vi "To Catalogue Cluster.vi"(8 "error in":errorcluster, 10 "Raw Catalogue":string="DEV:DB3.L1:LVL:DEV:MB1.T1:TEMP:DEV:DB7.G1:AUX:DEV:MB0.H1:HTR\n") -> (0 "error out":errorcluster, 1 "Devices":string[](array[string]), 2 "Catalouge":T1)   [LabVIEW 2015, in "Mercury iXX.lvlib"]
uses:
  Mercury iXX.lvlib
  Public/Libraries/System/Controls/Catalogue.ctl
  <vilib>/regexp/Match Regular Expression.xnode
  Public/Libraries/System.lvlib
panel:
  # "Mainboard"
  # "Daughter Boards"
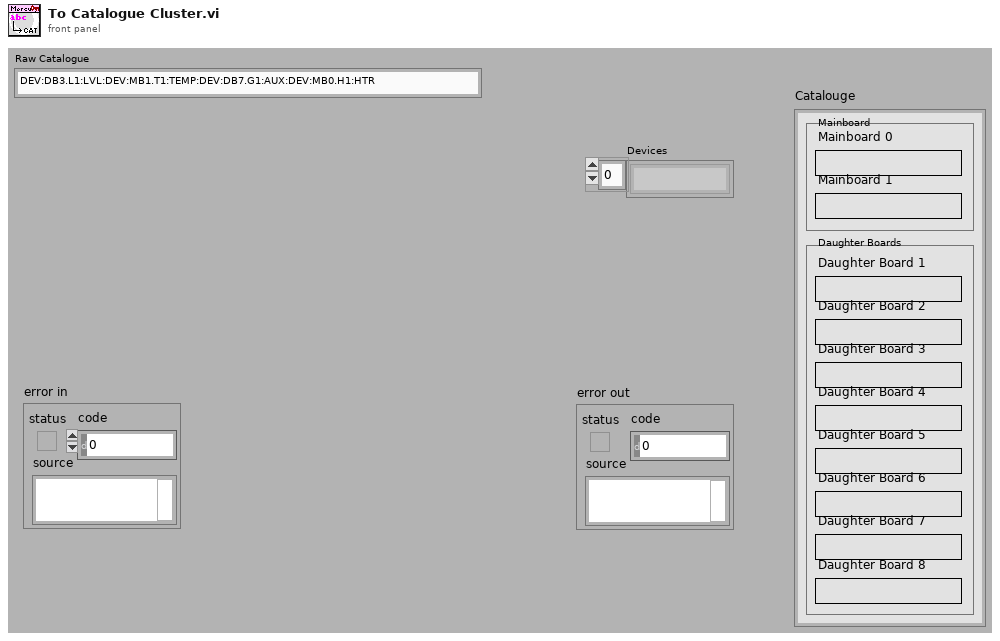
[diagram p1: front panel]
types:
  T1 = typedef "Mercury iXX.lvlib/System.lvlib/Catalogue.ctl" = cluster{"Mainboard 0":string, "Mainboard 1":string, "Daughter Board 1":string, "Daughter Board 2":string, "Daughter Board 3":string, "Daughter Board 4":string, "Daughter Board 5":string, "Daughter Board 6":string, "Daughter Board 7":string, "Daughter Board 8":string}
  T2 = cluster{"[0]":string, "[1]":string, "[2]":string, "[3]":string, "[4]":string, "[5]":string, "[6]":string, "[7]":string, "[8]":string, "[9]":string}
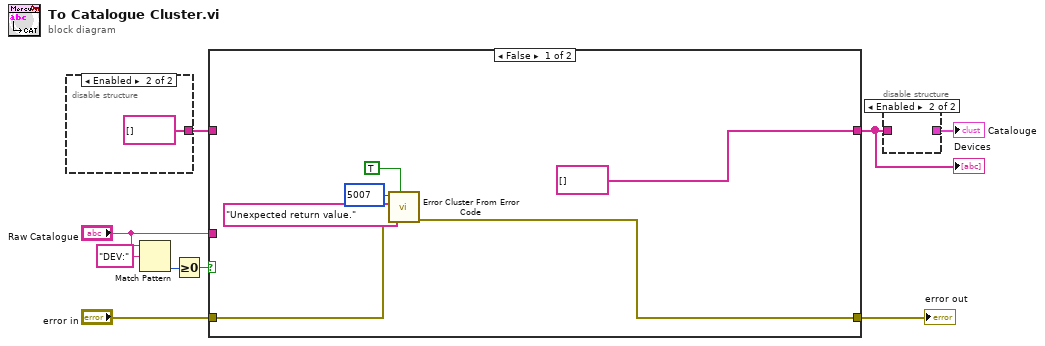
[diagram p0: block diagram]
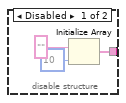
[diagram p2: hidden frame]
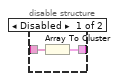
[diagram p3: hidden frame]
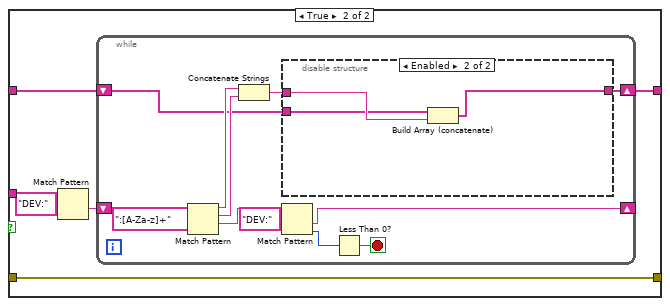
[diagram p4: hidden frame]
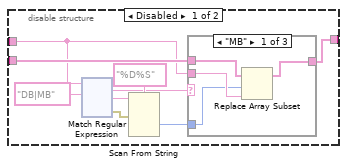
[diagram p5: hidden frame]
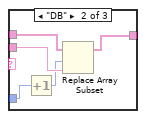
[diagram p6: hidden frame]
diagram:
  n1 = disable-structure shown="Enabled" {
    disable-tunnel: [w10 string[] []] -> w1
    frame Disabled {
      n2 = Initialize Array("", 10 ("dimension size")) -> (w10:string[])
    }
    frame Enabled {
    }
  }
  n3 = Match Pattern(string="Raw Catalogue", regular expression="DEV:") -> (offset past match=w9:i32)  [unwired: 4 out]
  n4 = Greater Or Equal To 0?(x=w9) -> (x >= 0?=w7:bool)
  n5 = case shown="False" w7 {
    tunnel: "Raw Catalogue" -> [_ w25]
    tunnel: [string[] [] w20] -> w3
    tunnel: [w18 w22] -> w6
    tunnel: "error in" -> [w14 w22]
    tunnel: w1 -> [_ w21]
    frame False {
      n6 = call <vilib>:"Error Cluster From Error Code.vi"("show call chain? (False)"=TRUE, "error in (no error)"=w14, "error message (\"\")"="Unexpected return value." ("error message (\"\")"), "error code (0)"=5007) -> ("error out"=w18:errorcluster)  [unwired: 5 out]
    }
    frame True {
      n7 = Match Pattern(string=w25, regular expression="DEV:") -> (after substring=w23:string)  [unwired: 4 out]
      n8 = while {
        shift-right: [w34] -> _
        shift-left: w23 -> [w37]
        shift-right: [w27] -> w20
        shift-left: w21 -> [w28]
        stop <- w32 stop-if-true
        n9 = Match Pattern(string=w37, regular expression=":[A-Za-z]+") -> (before substring=w30:string, match substring=w29:string, after substring=w35:string)  [unwired: 2 out]
        n10 = Concatenate Strings(w30, w29) -> (w26:string)
        n11 = Match Pattern(string=w35, regular expression="DEV:") -> (after substring=w34:string, offset past match=w33:i32)  [unwired: 3 out]
        n12 = disable-structure shown="Enabled" {
          disable-tunnel: w28 -> [w41 w172]
          disable-tunnel: [w40 w171] -> w27
          disable-tunnel: w26 -> [w39 w173]
          frame Disabled {
            n13 = xnode "Match Regular Expression"("input string"=w39, "regular expression"="DB|MB") -> ("whole match"=w42:string, "after match"=w44:string, "error out"=w45:errorcluster)  [unwired: 2 in, 4 out]
            n14 = Scan From String(format string="%D%S", input string=w44, error in=w45) -> (output 1=w38:i32)  [unwired: 1 in, 6 out]
            n15 = case shown="\"MB\"" w42 {
              tunnel: w41 -> [w50 w55 w56]
              tunnel: [w48 w52 w56] -> w40
              tunnel: w39 -> [w49 w54 _]
              tunnel: w38 -> [w47 w53 _]
              frame "MB" {
                n16 = Replace Array Subset(array=w50, new element=w49, index=w47) -> (w48:string[])
              }
              frame "DB" {
                n17 = Increment(x=w53) -> (x+1=w51:i32)
                n18 = Replace Array Subset(array=w55, new element=w54, index=w51) -> (w52:string[])
              }
              frame Default {
              }
            }
          }
          frame Enabled {
            n19 = Build Array (concatenate)(w172, w173) -> (w171:string[])
          }
        }
        n20 = Less Than 0?(x=w33) -> (x < 0?=w32:bool)
      }
    }
  }
  "error out" <- w6
  "Devices" <- w3
  n21 = disable-structure shown="Enabled" {
    disable-tunnel: w3 -> [w175 _]
    disable-tunnel: [w174 _] -> w2
    frame Disabled {
      n22 = Array To Cluster(array=w175) -> (cluster=w174:T2)
    }
    frame Enabled {
    }
  }
  "Catalouge" <- w2
